vi "SV TDMS Write Waveform (SGL) (1 Ch).vi"(0 "tdms file":refnum<k34>, 1 "write channel properties":bool=TRUE, 5 "group name in":string="Waveform", 7 "channel name in":string="Channel0", 9 "scaled signal [EU]":waveform(sgl), 11 "error in":errorcluster) -> (4 "tdms file out":refnum<k34>, 6 "group name out":string, 8 "channel name out":string, 15 "error out":errorcluster)   [LabVIEW 2017]
doc: "Writes data to the specified .tdms file in a format specific to the polymorphic instance. Wire data to the <B>scaled signal [EU]</B> input to determine the polymorphic instance to use or manually select the instance."
uses:
  <vilib>/addons/_NISVFA/_Shared subVIs/Controls/LV Datatypes.ctl
  <vilib>/addons/_NISVFA/_Shared subVIs/Controls/NI Function Type.ctl
  <vilib>/addons/_NISVFA/_Shared subVIs/Controls/NI Function SubType.ctl
  <vilib>/addons/_NISVFA/_Shared subVIs/Controls/svc_X-Axis Units.ctl
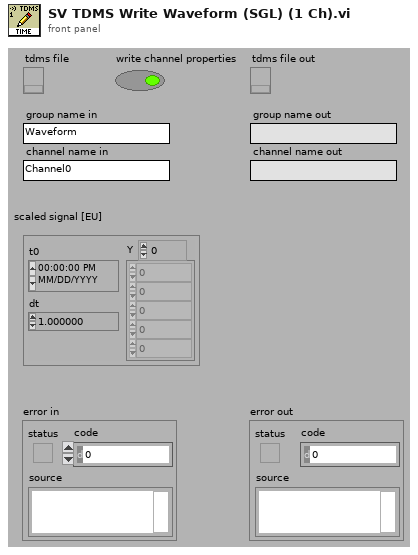
[diagram p1: front panel]
types:
  T1 = cluster{"X-axis label":string, "X-unit string":string, "Y-axis label":string, "Y-unit string":string}
  T2 = typedef "NI Function Type.ctl" = u16
  T3 = typedef "NI Function SubType.ctl" = u16
  T4 = typedef "svc_X-Axis Units.ctl" = u16
  T5 = cluster{"function type":T2, "function subtype":T3, "X-dimension":T4}
  T6 = typedef "LV Datatypes.ctl" = i32
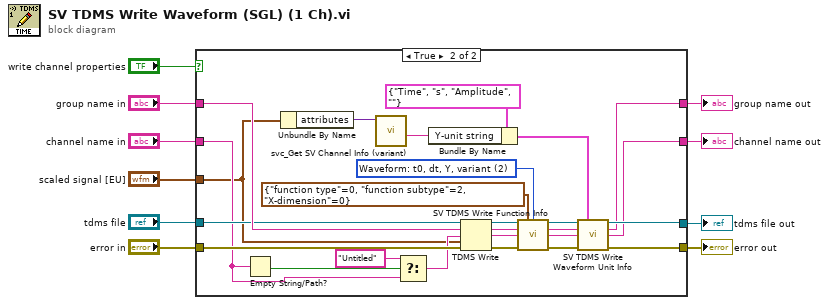
[diagram p0: block diagram]
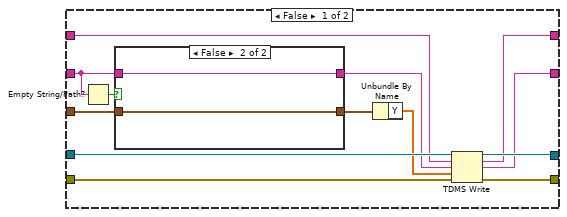
[diagram p2: hidden frame]
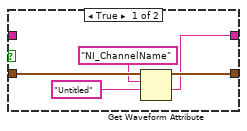
[diagram p3: hidden frame]
diagram:
  n1 = case shown="True" "write channel properties" {
    tunnel: [w18 w47] -> w10
    tunnel: [w13 w42] -> w9
    tunnel: "channel name in" -> [w23 w35]
    tunnel: "group name in" -> [w11 w56]
    tunnel: "tdms file" -> [w19 w55]
    tunnel: "scaled signal [EU]" -> [w21 w31]
    tunnel: [w17 w40] -> w4
    tunnel: [w16 w41] -> w3
    tunnel: "error in" -> [w12 w54]
    frame False {
      n2 = Empty String/Path?(string/path=w23) -> (empty?=w22:bool)
      n3 = case shown="False" w22 {
        tunnel: w23 -> [_ w29]
        tunnel: w21 -> [w28 w30]
        tunnel: [w27 w30] -> w20
        tunnel: [w24 w29] -> w14
        frame True {
          n4 = Get Waveform Attribute(5:"Untitled" ("t"), 6:"NI_ChannelName" ("name"), 7:w28) -> (1:w24:string, 3:w27:waveform(sgl))  [unwired: 1 in, 2 out]
        }
        frame False {
        }
      }
      n5 = Unbundle By Name(w20) -> ("Y"=w15:sgl[])
      n6 = TDMS Write(0:w19, 5:w11, 7:w14, 9:w15, 11:w12) -> (4:w18:refnum<k34>, 6:w17:string, 8:w16:string, 15:w13:errorcluster)  [unwired: 1 in]
    }
    frame True {
      w37 = T6 2 items=["String"=-2, "Boolean"=-1, "Scalar: y"=0, "Array: Y"=1, "Waveform: t0, dt, Y, variant"=2, "Cluster: x0, dx, Y"=3, "Cluster: X, Y"=4, "Waterfall"=5, "Colormap"=6] ("LabVIEW datatype")
      n7 = Empty String/Path?(string/path=w35) -> (empty?=w36:bool)
      n8 = Unbundle By Name(w31) -> ("attributes"=w32:variant)
      n9 = call <vilib>:"svc_Get SV Channel Info (variant).vi"("attributes"=w32) -> ("unit label"=w48:string)  [unwired: 5 in, 5 out]
      n10 = Select(t="Untitled", s=w36, f=w35) -> (s? t:f=w34:string)
      n11 = Bundle By Name(cluster=T1 {"X-axis label"="Time", "X-unit string"="s", "Y-axis label"="Amplitude", "Y-unit string"=""} ("unit info"), "Y-unit string"=w48) -> (w39:T1)
      n12 = TDMS Write(0:w55, 5:w56, 7:w34, 9:w31, 11:w54) -> (4:w46:refnum<k34>, 6:w45:string, 8:w44:string, 15:w43:errorcluster)  [unwired: 1 in]
      n13 = call <vilib>:"SV TDMS Write Function Info.vi"("tdms file in"=w46, "function info"=T5 {"function type"=0, "function subtype"=2, "X-dimension"=0}, "LabVIEW datatype"=w37, "group name"=w45, "channel name"=w44, "error in (no error)"=w43) -> ("tdms file out"=w53:refnum<k34>, "group name out"=w52:string, "channel name out"=w51:string, "error out"=w50:errorcluster)  [unwired: 6 in]
      n14 = call <vilib>:"SV TDMS Write Waveform Unit Info.vi"("tdms file"=w53, "unit info"=w39, "group name"=w52, "channel name"=w51, "error in (no error)"=w50) -> ("tdms file out"=w47:refnum<k34>, "group name out"=w40:string, "channel name out"=w41:string, "error out"=w42:errorcluster)  [unwired: 7 in]
    }
  }
  "tdms file out" <- w10
  "error out" <- w9
  "channel name out" <- w3
  "group name out" <- w4
